vi "Reset.vi"(8 "Error In":errorcluster, 11 "Thorlabs in":refnum<class "Thorlabs.lvclass">) -> (0 "Error Out":errorcluster, 3 "Thorlabs out":refnum<class "Thorlabs.lvclass">)   [LabVIEW 2018, in "Thorlabs.lvlib" / "Thorlabs.lvclass"]
doc: "This VI will reset the Motor/Actuator. This resets the stage to its default state, and closes and reopens the connection. This can be used when a bad state is entered.\n\nCreator: Slade Jeppesen\nCreated: 10/07/20"
uses:
  Thorlabs.lvclass
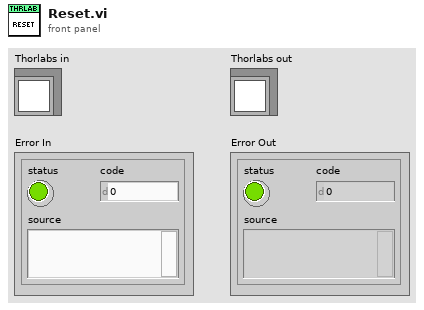
[diagram p1: front panel]
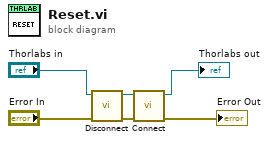
[diagram p0: block diagram]
diagram:
  n1 = call-dynamic "Disconnect.vi"("error in"="Error In", "Thorlabs In"="Thorlabs in") -> ("error out"=w5:errorcluster, "Thorlabs Out"=w3:refnum<class "Thorlabs.lvclass">)  [unwired: 8 in]
  n2 = call-dynamic "Connect.vi"("error in"=w5, "Thorlabs In"=w3) -> ("error out"=→"Error Out":errorcluster, "Thorlabs Out"=→"Thorlabs out":refnum<class "Thorlabs.lvclass">)  [unwired: 8 in]
